vi "Copy Async to Inline.vi"(8 "error in (no error)":errorcluster, 11 "Buffers in":refnum<class "Buffers.lvclass">) -> (0 "error out":errorcluster, 3 "Buffers out":refnum<class "Buffers.lvclass">)   [LabVIEW 2017, in "DSF Core.lvlib" / "Buffers.lvclass"]
uses:
  Buffers.lvclass
  Buffers.lvclass/Buffers.ctl
  <vilib>/NI/Memory Manager/Classes/Pointer/Pointer.lvclass/Pointer.ctl
  <vilib>/NI/Memory Manager/Classes/Pointer/Get Size.vi
  <vilib>/NI/Memory Manager/Classes/Pointer/Copy.vi
  <vilib>/NI/Memory Manager/Classes/Pointer/Copy (No Check).vi
  <vilib>/NI/Memory Manager/Classes/Pointer/Check Pointer Bounds.vi
  <vilib>/NI/Memory Manager/Classes/Pointer/Check Null Pointer.vi
  <vilib>/NI/Memory Manager/Classes/Pointer/Get Address.vi
  <vilib>/NI/Memory Manager/Classes/Pointer/Errors.vi
  <vilib>/NI/Memory Manager/Classes/Pointer/Out of Bounds.vi
  <vilib>/NI/Memory Manager/Classes/Pointer/Null Pointer.vi
  <vilib>/NI/Memory Manager/Classes/Pointer/Is Null.vi
  <vilib>/NI/Memory Manager/VIs/Source.Write.String.vi
  <vilib>/NI/Memory Manager/Classes/Pointer/Write Pointer Size.vi
  <vilib>/NI/Memory Manager/Classes/Pointer/Create Error.vi
  <vilib>/NI/Memory Manager/VIs/Source.Write.Scalar.Base10.vi
  <vilib>/NI/Memory Manager/VIs/Source.Write.Scalar.Base10 (U64).vi
  <vilib>/NI/Memory Manager/VIs/New Error Cluster Constant.vi
  <vilib>/NI/Memory Manager/VIs/New Error Cluster Constant (512B).vi
  <vilib>/NI/Memory Manager/VIs/Error Cluster.Set Status.vi
  <vilib>/NI/Memory Manager/VIs/Error Cluster.Set Code.vi
  <vilib>/NI/Memory Manager/VIs/Error Cluster.Set VI Source.vi
  <vilib>/NI/Memory Manager/Constants/Constants.vi
  <vilib>/NI/Memory Manager/Constants/Library Name.vi
  <vilib>/NI/Memory Manager/Classes/Pointer/Pointer Error Info.vi
  <vilib>/NI/Memory Manager/Constants/Pointer Class Name.vi
  Buffer.lvclass
  C:/Program Files (x86)/National Instruments/LabVIEW 2017/vi.lib/NI/Memory Manager/Classes/Pointer/Pointer.lvclass
  <vilib>/NI/Memory Manager/Classes/Pointer/Pointer.lvclass
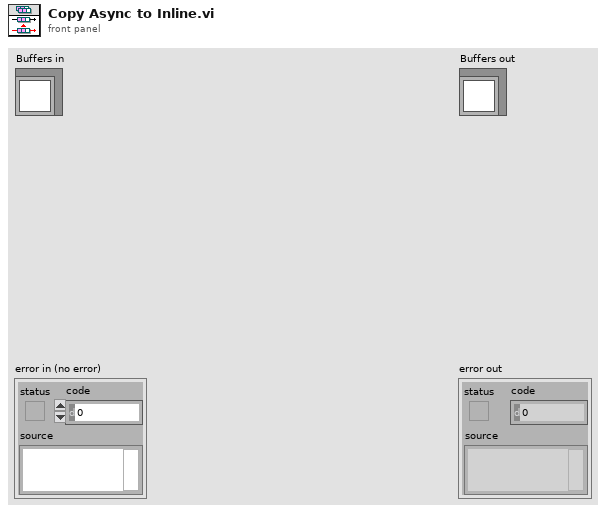
[diagram p1: front panel]
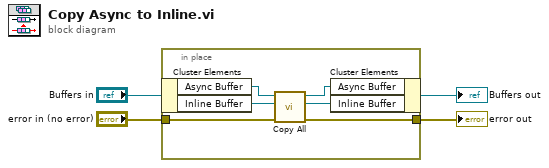
[diagram p0: block diagram]
diagram:
  n1 = in-place {
    in-place-border: "error in (no error)" -> [w8]
    in-place-border: [w7] -> w2
    n2 = in-place-cluster #1("Buffers in") -> ("Async Buffer"=w9:refnum<class "Buffer.lvclass">, "Inline Buffer"=w10:refnum<class "Buffer.lvclass">)
    n3 = call <vilib>:"Copy All.vi"("error in (no error)"=w8, "dst Pointer in"=w10, "src Pointer in"=w9) -> ("error out"=w7:errorcluster, "dst Pointer out"=w6:refnum<class "Buffer.lvclass">, "src Pointer out"=w5:refnum<class "Buffer.lvclass">)  [unwired: 6 in]
    n4 = in-place-cluster #1("Async Buffer"=w5, "Inline Buffer"=w6) -> (→"Buffers out":refnum<class "Buffers.lvclass">)
  }
  "error out" <- w2
